vi "SVXMPL_Build Orbit PLot (WDT).vi"(8 "error in (no error)":errorcluster, 10 "Ch B":waveform(dbl)={"t0"=timestamp(0 s since 1904-01-01), "dt"=0.0, "Y"=[]}, 11 "Ch A":waveform(dbl)={"t0"=timestamp(0 s since 1904-01-01), "dt"=0.0, "Y"=[]}) -> (0 "error out":errorcluster, 3 "Orbit Plot":cluster{"Y":dbl[], "Y":dbl[]}(graph))   [LabVIEW 2017]
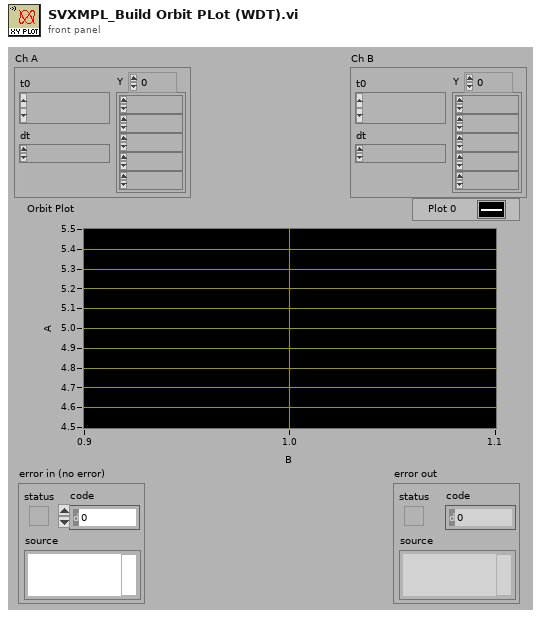
[diagram p1: front panel]
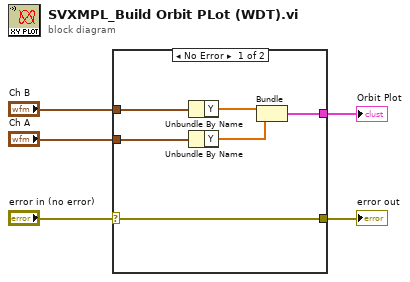
[diagram p0: block diagram]
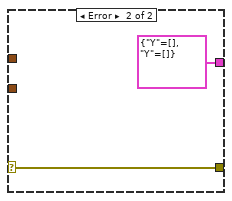
[diagram p2: hidden frame]
diagram:
  n1 = case shown="No Error" "error in (no error)" {
    selector: "error in (no error)" -> [w6 w13]
    tunnel: [w11 cluster{"Y":dbl[], "Y":dbl[]} {"Y"=[], "Y"=[]}] -> w5
    tunnel: "Ch B" -> [w8 _]
    tunnel: "Ch A" -> [w7 _]
    tunnel: [w6 w13] -> w1
    frame No Error {
      n2 = Unbundle By Name(w8) -> ("Y"=w9:dbl[])
      n3 = Unbundle By Name(w7) -> ("Y"=w10:dbl[])
      n4 = Bundle("Y"=w9, "Y"=w10) -> (w11:cluster{"Y":dbl[], "Y":dbl[]})  [unwired: 1 in]
    }
    frame Error {
    }
  }
  "Orbit Plot" <- w5
  "error out" <- w1
